vi "Get Request ID.vi"(8 "error in (no error)":errorcluster, 11 "Request in":refnum<class "Request.lvclass">) -> (0 "error out":errorcluster, 2 "Request ID":string, 3 "Request out":refnum<class "Request.lvclass">)   [LabVIEW 2020, in "obs-websocket.lvlib" / "Request.lvclass"]
uses:
  Request.lvclass
  Request.lvclass/Request.ctl
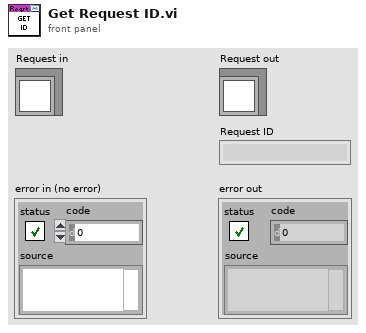
[diagram p1: front panel]
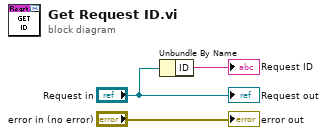
[diagram p0: block diagram]
diagram:
  n1 = Unbundle By Name("Request in") -> ("ID"=→"Request ID":string)
  "error out" <- "error in (no error)"
  "Request out" <- "Request in"
